vi "Plot.vi"(8 "error in (no error)":errorcluster, 11 "Spectrum Recorder in":refnum<class "Spectrum Recorder too.lvclass">) -> (0 "error out":errorcluster, 3 "Spectrum Recorder out":refnum<class "Spectrum Recorder too.lvclass">)   [LabVIEW 2016, in "Spectrum Recorder too.lvclass"]
uses:
  Spectrum Recorder too.lvclass
  Spectrum Recorder too.lvclass/Spectrum Recorder too.ctl
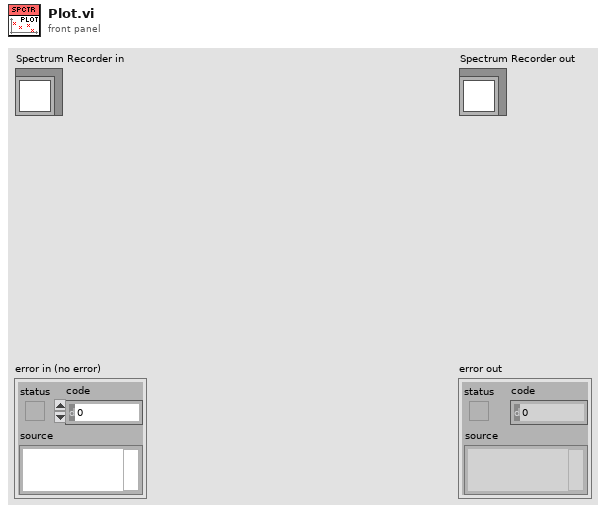
[diagram p1: front panel]
types:
  T1 = enum16{"open", "open or create", "create or replace", "create", "open (read-only)"}
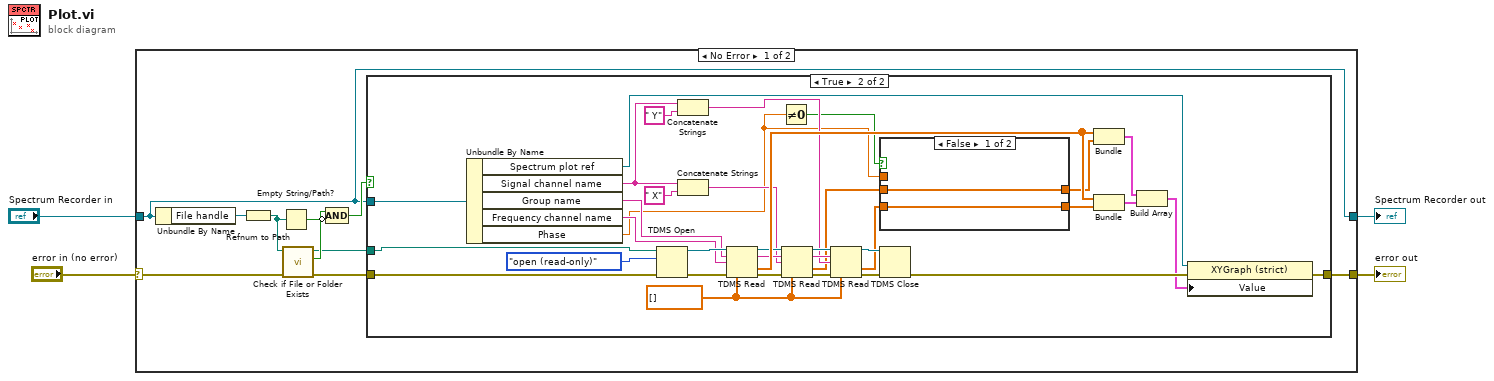
[diagram p0: block diagram]
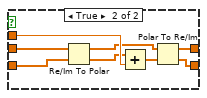
[diagram p3: hidden frame]
diagram:
  n1 = case shown="No Error" "error in (no error)" {
    selector: "error in (no error)" -> [w8 w62]
    tunnel: [w7 w62] -> w3
    tunnel: [w9 w61] -> w1
    tunnel: "Spectrum Recorder in" -> [w9 w61]
    frame No Error {
      n2 = Unbundle By Name(w9) -> ("File handle"=w6:refnum<k34>)
      n3 = Refnum to Path(1:w6) -> (0:w5:path)
      n4 = Empty String/Path?(string/path=w5) -> (empty?=w13:bool)
      n5 = call <vilib>:"Check if File or Folder Exists.vi"("error in (no error)"=w8, "path"=w5) -> ("error out"=w10:errorcluster, "file or folder exists?"=w14:bool, "dup path"=w11:path)  [unwired: 7 in]
      n6 = Compound Arithmetic op=AND(w14, invert w13) -> (w12:bool)
      n7 = case shown="True" w12 {
        tunnel: w11 -> [_ w48]
        tunnel: w10 -> [w15 w47]
        tunnel: w9 -> [_ w45]
        tunnel: [w15 w41] -> w7
        frame False {
        }
        frame True {
          w24 = dbl[] []
          n8 = Unbundle By Name(w45) -> ("Spectrum plot ref"=w40:refnum<vi>, "Signal channel name"=w21:string, "Group name"=w44:string, "Frequency channel name"=w43:string, "Phase"=w17:dbl)
          n9 = TDMS Open(8:w47, 10:T1."open (read-only)" ("operation (0:open)"), 11:w48) -> (0:w49:errorcluster, 3:w50:refnum<k34>)  [unwired: 4 in]
          n10 = Concatenate Strings(w21, " Y" ("string")) -> (w20:string)
          n11 = Concatenate Strings(w21, " X" ("string")) -> (w22:string)
          n12 = TDMS Read(0:w50, 5:w44, 7:w43, 11:w49, 12:w24) -> (4:w35:refnum<k34>, 6:w33:string, 10:w36:dbl[], 15:w34:errorcluster)  [unwired: 3 in, 2 out]
          n13 = Not Equal To 0?(x=w17) -> (x != 0?=w16:bool)
          n14 = TDMS Read(0:w35, 5:w33, 7:w22, 11:w34, 12:w24) -> (4:w26:refnum<k34>, 6:w23:string, 10:w19:dbl[], 15:w28:errorcluster)  [unwired: 3 in, 2 out]
          n15 = TDMS Read(0:w26, 5:w23, 7:w20, 11:w28, 12:w24) -> (4:w25:refnum<k34>, 10:w18:dbl[], 15:w27:errorcluster)  [unwired: 3 in, 3 out]
          n16 = case shown="False" w16 {
            tunnel: w17 -> [_ w59]
            tunnel: [w52 w58] -> w32
            tunnel: [w51 w57] -> w31
            tunnel: w19 -> [w52 w56]
            tunnel: w18 -> [w51 w55]
            frame False {
            }
            frame True {
              n17 = Re/Im To Polar(2:w55, 3:w56) -> (0:w54:dbl[], 1:w53:dbl[])
              n18 = Add(x=w54, y=w59) -> (x+y=w60:dbl[])
              n19 = Polar To Re/Im(2:w60, 3:w53) -> (0:w57:dbl[], 1:w58:dbl[])
            }
          }
          n20 = TDMS Close(8:w27, 11:w25) -> (0:w42:errorcluster)  [unwired: 1 out]
          n21 = Bundle(w36, w32) -> (w39:cluster{dbl[], dbl[]})  [unwired: 1 in]
          n22 = Bundle(w36, w31) -> (w38:cluster{dbl[], dbl[]})  [unwired: 1 in]
          n23 = Build Array(w39, w38) -> (w37:cluster{dbl[], dbl[]}[])
          n24 = property class="XYGraph (strict)"(reference=w40, error in=w42, "Value"=w37) -> (error out=w41:errorcluster)  [unwired: 1 out]
        }
      }
    }
    frame Error {
    }
  }
  "error out" <- w3
  "Spectrum Recorder out" <- w1
